vi "ReadMarker.vi"(1 "MarkerIdx":i32, 2 "Data":u8[](array[numeric])) -> (0 "Marker":sgl[](array[numeric]))   [LabVIEW 2011]
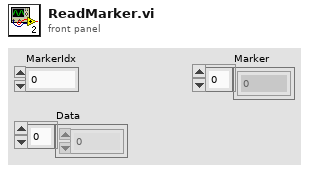
[diagram p1: front panel]
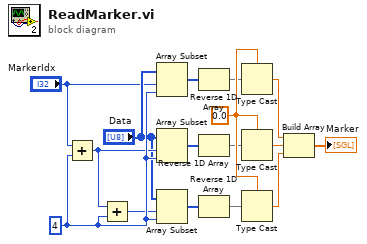
[diagram p0: block diagram]
diagram:
  w12 = sgl 0.0
  w8 = 4 ("length")
  n1 = Add(x="MarkerIdx", y=w8) -> (x+y=w6:i32)
  n2 = Add(x=w6, y=w8) -> (x+y=w7:i32)
  n3 = Array Subset(array="Data", index="MarkerIdx", length=w8) -> (w9:u8[])
  n4 = Array Subset(array="Data", index=w6, length=w8) -> (w10:u8[])
  n5 = Array Subset(array="Data", index=w7, length=w8) -> (w11:u8[])
  n6 = Reverse 1D Array(array=w9) -> (reversed array=w4:u8[])
  n7 = Reverse 1D Array(array=w10) -> (reversed array=w3:u8[])
  n8 = Reverse 1D Array(array=w11) -> (reversed array=w2:u8[])
  n9 = Type Cast(type=w12, x=w4) -> (*(type *) &x=w13:sgl)
  n10 = Type Cast(type=w12, x=w3) -> (*(type *) &x=w14:sgl)
  n11 = Type Cast(type=w12, x=w2) -> (*(type *) &x=w15:sgl)
  n12 = Build Array(w13, w14, w15) -> (→"Marker":sgl[])
